vi "DSF.Engine.Memory.BufferPool.Return Buffer.vi"(8 "error in (no error)":errorcluster, 9 "timeout ms (0)":i32 format="%d ms", 10 "Buffer":refnum<class "DSF.Engine.Memory.Buffer.lvclass">, 11 "BufferPool in":refnum<class "DSF.Engine.Memory.BufferPool.lvclass">) -> (0 "error out":errorcluster, 1 "timed out?":bool, 3 "BufferPool out":refnum<class "DSF.Engine.Memory.BufferPool.lvclass">)   [LabVIEW 2016, in "DSF.Engine.lvlib" / "DSF.Engine.Memory.BufferPool.lvclass"]
uses:
  BufferPool/DSF.Engine.Memory.BufferPool.lvclass
  Buffer/DSF.Engine.Memory.Buffer.lvclass
  Buffer/DSF.Engine.Memory.Buffer.lvclass/DSF.Engine.Memory.Buffer.ctl
  BufferPool/DSF.Engine.Memory.BufferPool.lvclass/DSF.Engine.Memory.BufferPool.ctl
  Memory.Buffer/Methods/DSF.Engine.Memory.Buffer.Errors.vi
  Memory.Buffer/Methods/DSF.Engine.Memory.Buffer.Errors.Invalid Buffer.vi
  Submodules/Memory Manager/Source/Submodules/SEH/Source/VIs/Static Error Handling.Error Cluster Constant.vi
  Submodules/Memory Manager/Source/Submodules/SEH/Source/VIs/Static Error Handling.Error Cluster Constant (512B).vi
  Submodules/Memory Manager/Source/Submodules/SEH/Source/VIs/Static Error Handling.Parameters.Status.Set.vi
  Submodules/Memory Manager/Source/Submodules/SEH/Source/VIs/Static Error Handling.Parameters.VI Source.Set.vi
  Constants/DSF.Shared.Constants.vi
  Constants/DSF.Shared.Constants.Library Name.vi
  Submodules/Memory Manager/Source/Submodules/SEH/Source/VIs/Static Error Handling.Parameters.Code.Set.vi
  Submodules/Memory Manager/Source/Submodules/SEH/Source/VIs/Static Error Handling.Source Buffer.Write.String.vi
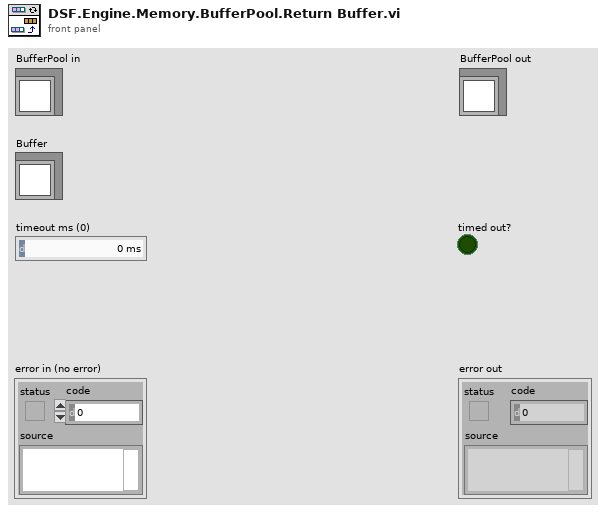
[diagram p1: front panel]
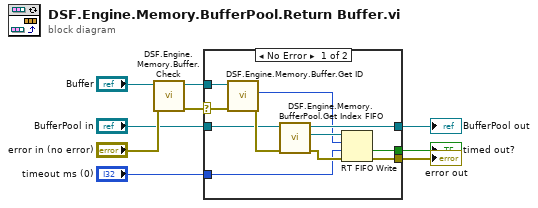
[diagram p0: block diagram]
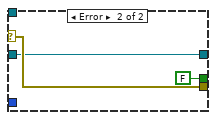
[diagram p2: hidden frame]
diagram:
  n1 = call "DSF.Engine.Memory.Buffer.Check.vi"("error in (no error)"="error in (no error)", "Buffer in"="Buffer") -> ("error out"=w1:errorcluster, "Buffer out"=w4:refnum<class "DSF.Engine.Memory.Buffer.lvclass">)  [unwired: 8 in]
  n2 = case shown="No Error" w1 {
    selector: w1 -> [w10 w23]
    tunnel: "timeout ms (0)" -> [w18 _]
    tunnel: [w17 w22] -> w8
    tunnel: [w16 w23] -> w7
    tunnel: [w15 FALSE ("timed out?")] -> w6
    tunnel: w4 -> [w12 _]
    tunnel: "BufferPool in" -> [w11 w22]
    frame No Error {
      n3 = call "DSF.Engine.Memory.Buffer.Get ID.vi"("error in (no error)"=w10, "Buffer in"=w12) -> ("error out"=w13:errorcluster, "id"=w14:i32)  [unwired: 7 in, 1 out]
      n4 = call "DSF.Engine.Memory.BufferPool.Get Index FIFO.vi"("error in (no error)"=w13, "BufferPool in"=w11) -> ("error out"=w19:errorcluster, "Index FIFO"=w20:refnum<k33>, "BufferPool out"=w17:refnum<class "DSF.Engine.Memory.BufferPool.lvclass">)  [unwired: 7 in]
      n5 = RT FIFO Write(0:w20, 1:w14, 2:w18, 3:w19) -> (10:w15:bool, 11:w16:errorcluster)  [unwired: 1 in, 2 out]
    }
    frame Error {
    }
  }
  "error out" <- w7
  "BufferPool out" <- w8
  "timed out?" <- w6
